vi "Adjust_Image_Quality.vi"() -> ()   [LabVIEW 2017]
uses:
  <vilib>/userdefined/High Color/IMAQdx.ctl
  <vilib>/vision/driver/NI_Vision_Acquisition_Software.lvlib
panel:
  out "Histogram Graph":cluster{dbl[], dbl[]}(graph)
  in  "Slide":dbl(slide) scale=0.0..1.0
  in  "Brightness":i64(slide) scale=0.0..255.0
  in  "stop":bool
  out "Standard  Variation":sgl
  out "Mean Value":sgl
  out "Range":sgl
  out "Within Range":bool
  out "Image":T1(plugin-control)
  out "error out":errorcluster
  in  "Session In":T2
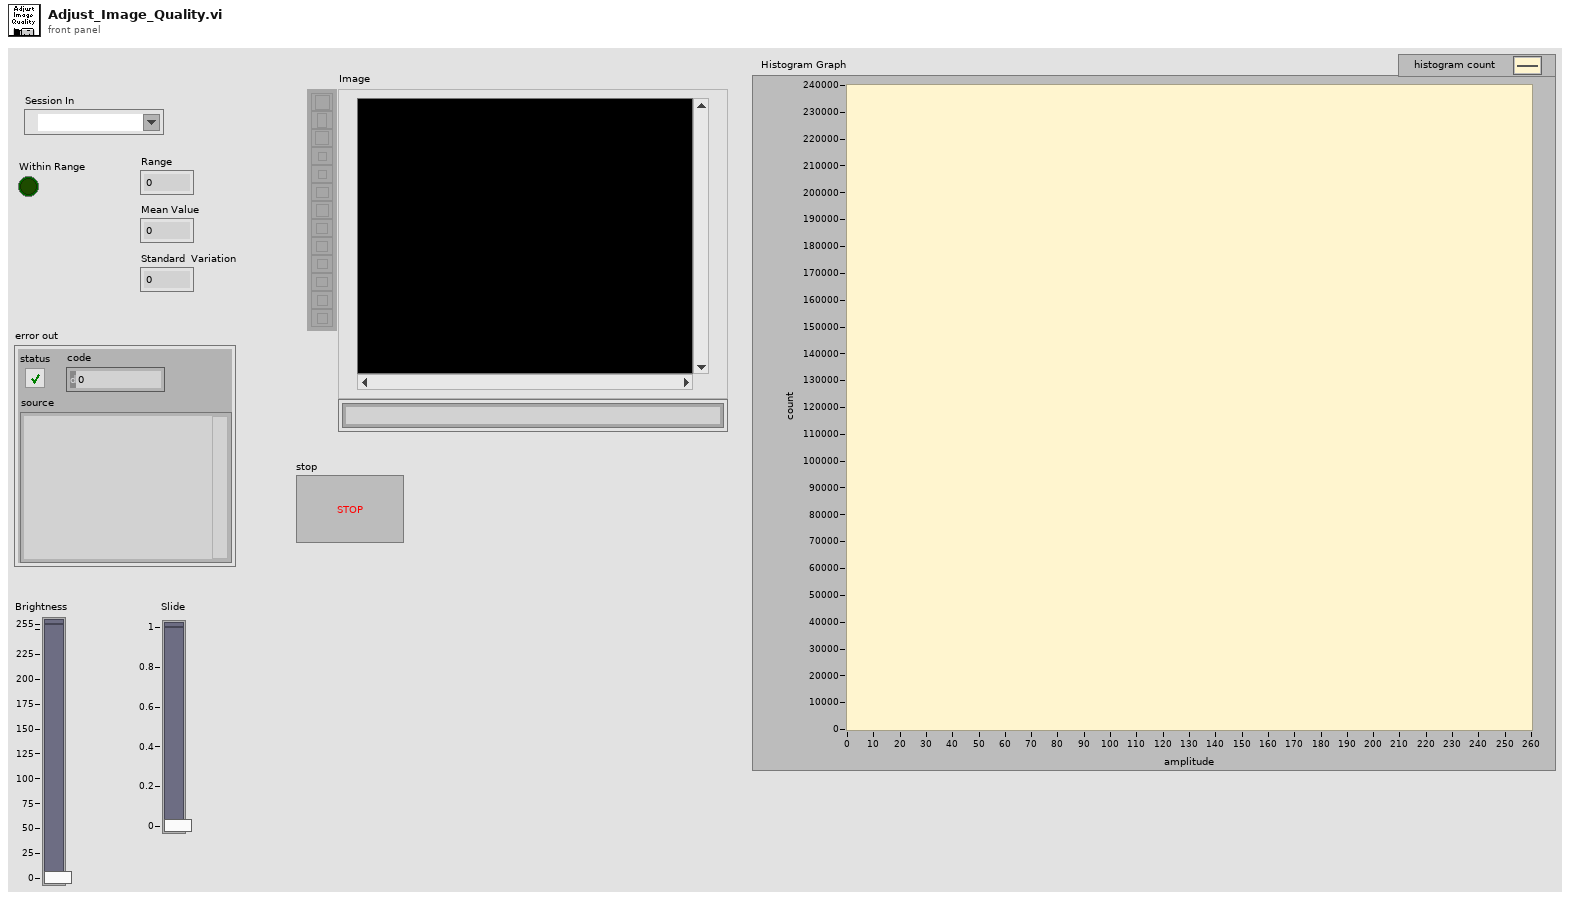
[diagram p1: front panel]
types:
  T1 = typedef "IMAQ Image.ctl" = refnum<image>
  T2 = typedef "IMAQdx.ctl" = refnum<k21>
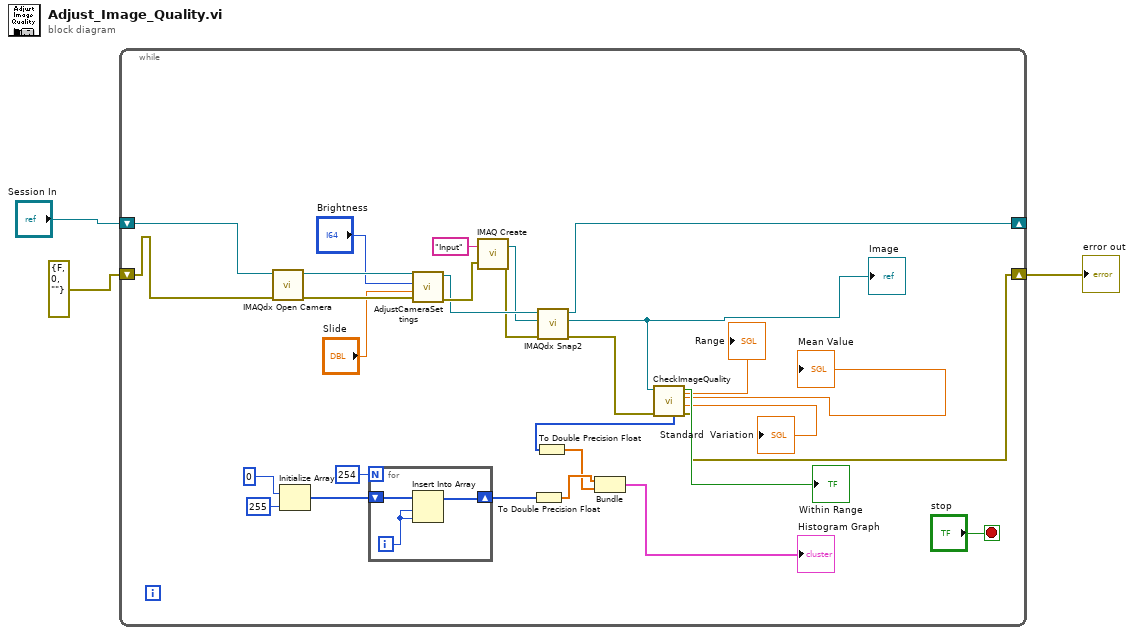
[diagram p0: block diagram]
diagram:
  n1 = while {
    shift-right: [w18] -> _
    shift-left: "Session In" -> [w19]
    shift-right: [w15] -> w1
    shift-left: errorcluster {"status"=FALSE, "code"=0, "source"=""} ("error out") -> [w20]
    stop <- "stop" stop-if-true
    n2 = call <vilib>:"IMAQdx Open Camera.vi"("error in"=w20, "Session In"=w19) -> ("error out"=w29:errorcluster, "Session Out"=w28:T2)  [unwired: 8 in]
    n3 = Initialize Array(0, 255 ("dimension size")) -> (w9:i32[])
    n4 = for {
      N: 254 -> [_]
      shift-right: [w33] -> w7
      shift-left: w9 -> [w34]
      i -> [w35]
      n5 = Insert Into Array(array=w34, index=w35, new element=w35) -> (w33:i32[])
    }
    n6 = call "AdjustCameraSettings.vi"("error in (no error)"=w29, "Contrast"="Slide", "Brightness"="Brightness", "Session In"=w28) -> ("error out"=w31:errorcluster, "IMAQdx Session"=w30:T2)  [unwired: 4 in, 2 out]
    n7 = call "IMAQ Create"("Image Name"="Input", "error in (no error)"=w31) -> ("New Image"=w22:T1, "error out"=w23:errorcluster)  [unwired: 3 in]
    n8 = To Double Precision Float(number=w7) -> (double precision float=w5:dbl[])
    n9 = call <vilib>:"IMAQdx Snap2.vi"("error in"=w23, "Image In"=w22, "Session In"=w30) -> ("error out"=w24:errorcluster, "Image Out"=w16:T1, "Session Out"=w18:T2)  [unwired: 6 in]
    "Image" <- w16
    n10 = call "CheckImageQuality.vi"("error in (no error)"=w24, "Image"=w16) -> ("error out"=w15:errorcluster, "Standard  Variation"=→"Standard  Variation":sgl, "Mean Value"=→"Mean Value":sgl, "Within Range"=→"Within Range":bool, "histogram"=w12:u32[], "Range"=→"Range":sgl)  [unwired: 4 in]
    n11 = To Double Precision Float(number=w12) -> (double precision float=w4:dbl[])
    n12 = Bundle(w5, w4) -> (→"Histogram Graph":cluster{dbl[], dbl[]})  [unwired: 1 in]
  }
  "error out" <- w1
